vi "init_valve.vi"(8 "error in":errorcluster) -> (0 "error out":errorcluster)   [LabVIEW 2013]
uses:
  <vilib>/Utility/config.llb/Read Key (String).vi
  <vilib>/Utility/config.llb/Read Key (U32).vi
  <vilib>/Utility/config.llb/NI_LVConfig.lvlib
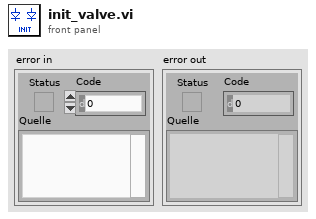
[diagram p1: front panel]
types:
  T1 = cluster{"Mode":enum16{"RTU", "ASCII"}, "Slave Address":u8}
  T2 = typedef "NI_LVConfig.lvlib/Config Data RefNum.ctl" = refnum<k1>
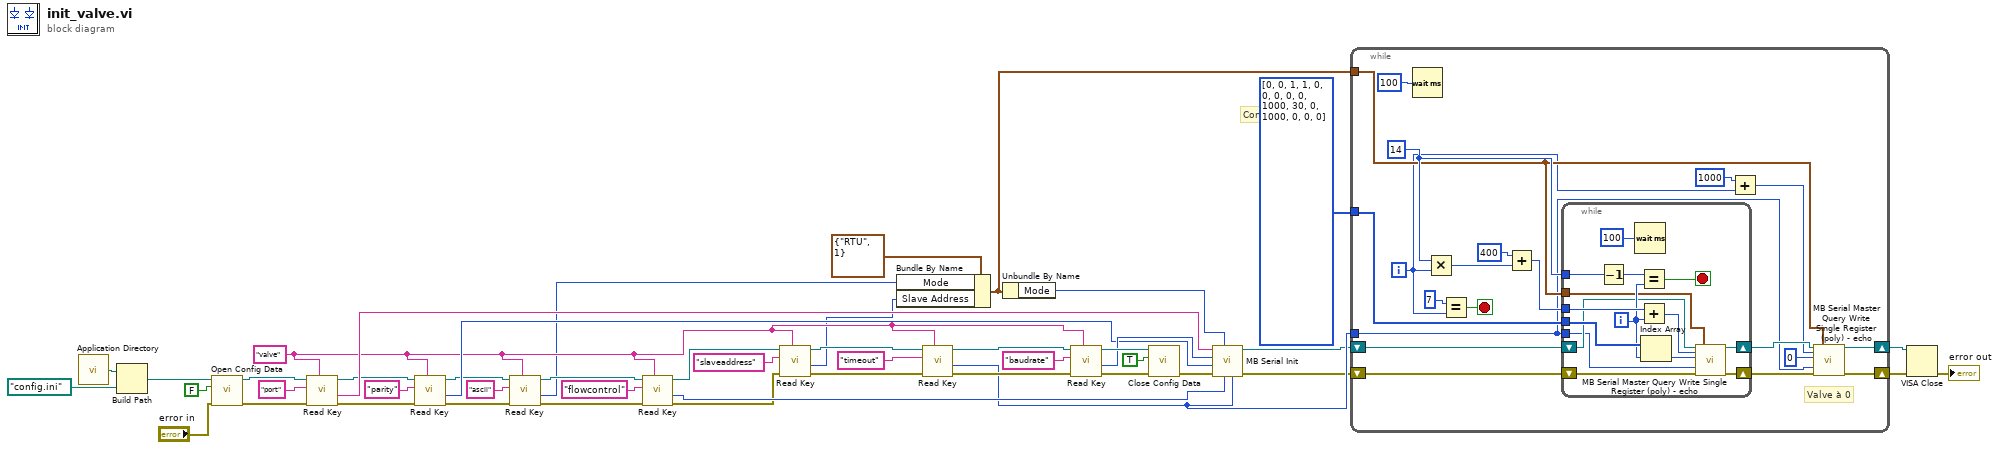
[diagram p0: block diagram]
diagram:
  w12 = "valve" ("section")
  # "Config"
  n1 = call <vilib>:"Application Directory.vi"() -> ("Application Directory"=w39:path)
  n2 = Build Path(base path=w39, name or relative path=path "config.ini" ("default name")) -> (appended path=w43:path)
  n3 = call <vilib>:"Open Config Data.vi"("error in (no error)"="error in", "create file if necessary (T)"=FALSE ("create file if necessary? (T)"), "configuration file path"=w43) -> ("error out"=w42:errorcluster, "refnum"=w40:T2)  [unwired: 6 in, 1 out]
  n4 = call-poly <vilib>:"Read Key.vi"("section"=w12, "error in (no error)"=w42, "key"="port", "refnum"=w40) -> ("error out"=w26:errorcluster, "value"=w28:string, "refnum out"=w25:T2)  [unwired: 4 in, 1 out]
  n5 = call-poly <vilib>:"Read Key.vi"("section"=w12, "error in (no error)"=w26, "key"="parity", "refnum"=w25) -> ("error out"=w21:errorcluster, "value"=w24:u32, "refnum out"=w18:T2)  [unwired: 4 in, 1 out]
  n6 = call-poly <vilib>:"Read Key.vi"("section"=w12, "error in (no error)"=w21, "key"="ascii", "refnum"=w18) -> ("error out"=w20:errorcluster, "value"=w10:u32, "refnum out"=w19:T2)  [unwired: 4 in, 1 out]
  n7 = call-poly <vilib>:"Read Key.vi"("section"=w12, "error in (no error)"=w20, "key"="flowcontrol", "refnum"=w19) -> ("error out"=w16:errorcluster, "value"=w22:u32, "refnum out"=w13:T2)  [unwired: 4 in, 1 out]
  n8 = call-poly <vilib>:"Read Key.vi"("section"=w12, "error in (no error)"=w16, "key"="slaveaddress", "refnum"=w13) -> ("error out"=w15:errorcluster, "value"=w9:u32, "refnum out"=w14:T2)  [unwired: 4 in, 1 out]
  n9 = Bundle By Name(cluster=T1 {"Mode"=enum."RTU", "Slave Address"=1} ("Serial Parameters"), "Mode"=w10, "Slave Address"=w9) -> (w7:T1)
  n10 = call-poly <vilib>:"Read Key.vi"("section"=w12, "error in (no error)"=w15, "key"="timeout", "refnum"=w14) -> ("error out"=w34:errorcluster, "value"=w6:u32, "refnum out"=w37:T2)  [unwired: 4 in, 1 out]
  n11 = Unbundle By Name(w7) -> ("Mode"=w47:enum16{"RTU", "ASCII"})
  n12 = call-poly <vilib>:"Read Key.vi"("section"=w12, "error in (no error)"=w34, "key"="baudrate", "refnum"=w37) -> ("error out"=w35:errorcluster, "value"=w29:u32, "refnum out"=w36:T2)  [unwired: 4 in, 1 out]
  n13 = call <vilib>:"Close Config Data.vi"("error in (no error)"=w35, "write file if changed (T)"=TRUE ("write configuration file? (T)"), "refnum"=w36) -> ("error out"=w31:errorcluster)  [unwired: 8 out]
  n14 = call "MB Serial Init.vi"("Timeout"=w6, "Flow Control"=w22, "Mode"=w47, "error in (no error)"=w31, "Parity"=w24, "Baud Rate"=w29, "VISA resource name"=w28) -> ("error out"=w2:errorcluster, "VISA resource name out"=w1:refnum<visa-resource-name>)  [unwired: 3 out]
  n15 = while {
    tunnel: w7 -> [w53]
    tunnel: w6 -> [w52]
    tunnel: i32[] [0, 0, 1, 1, 0, 0, 0, 0, 0, 1000, 30, 0, 1000, 0, 0, 0] -> [w65]
    shift-right: [w56] -> w4
    shift-left: w2 -> [w60]
    shift-right: [w57] -> w5
    shift-left: w1 -> [w59]
    i -> [w49]
    stop <- w66 stop-if-true
    w63 = 14
    # "Valve à 0"
    n16 = Wait (ms)(milliseconds to wait=100) -> ()  [unwired: 1 out]
    n17 = Multiply(x=w63, y=w49) -> (x*y=w62:i32)
    n18 = Equal?(x=7, y=w49) -> (x = y?=w66:bool)
    n19 = Add(x=400, y=w62) -> (x+y=w61:i32)
    n20 = while {
      tunnel: w53 -> [w73]
      tunnel: w52 -> [w68]
      tunnel: w65 -> [w81]
      tunnel: w63 -> [w80]
      tunnel: w61 -> [w78]
      shift-right: [w75] -> w55
      shift-left: w60 -> [w69]
      shift-right: [w74] -> w54
      shift-left: w59 -> [w70]
      i -> [w77]
      stop <- w82 stop-if-true
      n21 = Decrement(x=w80) -> (x-1=w79:i32)
      n22 = Wait (ms)(milliseconds to wait=100) -> ()  [unwired: 1 out]
      n23 = Equal?(x=w79, y=w77) -> (x = y?=w82:bool)
      n24 = Add(x=w78, y=w77) -> (x+y=w72:i32)
      n25 = Index Array(array=w81, index=w77) -> (element=w71:i32)
      n26 = call "MB Serial Master Query Write Single Register (poly) - echo.vi"("VISA resource name"=w70, "Address"=w72, "Holding Register"=w71, "Timeout"=w68, "error in"=w69, "Serial Parameters"=w73) -> ("VISA resource name out"=w74:refnum<visa-resource-name>, "error out"=w75:errorcluster)  [unwired: 11 in, 1 out]
    }
    n27 = Add(x=1000, y=w49) -> (x+y=w48:i32)
    n28 = call "MB Serial Master Query Write Single Register (poly) - echo.vi"("VISA resource name"=w54, "Address"=w48, "Holding Register"=0, "Timeout"=w52, "error in"=w55, "Serial Parameters"=w53) -> ("VISA resource name out"=w57:refnum<visa-resource-name>, "error out"=w56:errorcluster)  [unwired: 11 in, 1 out]
  }
  n29 = VISA Close(VISA resource name=w5, error in (no error)=w4) -> (error out=→"error out":errorcluster)
